vi "DigSeqLogic_Edge_On.vi"(11 "Input":bool) -> (3 "On Edge":bool)   [LabVIEW 2019, in "Trajectory_Library.lvlib"]
uses:
  Trajectory_Library.lvlib
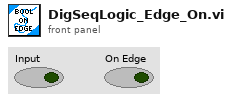
[diagram p1: front panel]
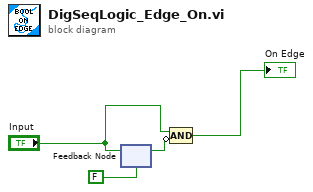
[diagram p0: block diagram]
diagram:
  n1 = feedback #1(FALSE ("Request")) -> (w2:bool)
  n2 = feedback-in #1("Input") -> ()
  n3 = Compound Arithmetic op=AND("Input", invert w2) -> (→"On Edge":bool)
